vi "SPD.QE&TR Meas.vi"(5 "Progress":refnum<vi>, 6 "Temperature index":i32, 7 "Continue":refnum<vi>, 8 "Error In":errorcluster, 10 "Already done":bool, 11 "SPD.Stand Ctrl in":T1 {"spdDeviceSession"."hidSPD.Sturtup Values"."HV_bias" format="%#_6p, V"; "spdDeviceSession"."hidSPD.Sturtup Values"."TSet" format="%#_6p, DegC"; "spdDeviceSession"."hidSPD.Controller"."HV_bias" format="%#_6p, V"; "spdDeviceSession"."hidSPD.Controller"."TSet" format="%#_6p, DegC"}) -> (0 "Error Out":errorcluster, 1 "pass":bool, 2 "Report":string, 3 "SPD.Stand Ctrl out":T1 {"spdDeviceSession"."hidSPD.Sturtup Values"."HV_bias" format="%#_6p, V"; "spdDeviceSession"."hidSPD.Sturtup Values"."TSet" format="%#_6p, DegC"; "spdDeviceSession"."hidSPD.Controller"."HV_bias" format="%#_6p, V"; "spdDeviceSession"."hidSPD.Controller"."TSet" format="%#_6p, DegC"})   [LabVIEW 2018]
uses:
  typedefs/SPD.Stand Ctrl.ctl
  Instruments/SPD HID Interface/hidSPDLibForLabView/LibVIs/hidSPD Controls/hidSPD Device Session.ctl
  Instruments/SPD HID Interface/hidSPDLibForLabView/LibVIs/hidSPD Controls/hidSPD Controller.ctl
  Instruments/SPD HID Interface/hidSPDLibForLabView/LibVIs/hidSPD Controls/hidSPD SPD Type.ctl
  Instruments/KC705 DevBoard/typedefs/DevB.Session.ctl
  Instruments/KeySight 53230A/typedefs/FreqC.Session.ctl
  Instruments/KeySight 8164B/KeySight 8164B LAN InstrLib/typedefs/KeySight 8164B control.ctl
  Instruments/LeCroy SDA830/typedefs/LeCroy.Session.ctl
  typedefs/SPD.Events.ctl
  ConfigFile/SPD.Config File ctrl.ctl
  <vilib>/Utility/config.llb/Config Data RefNum.ctl
  typedefs/SPD.Meas Result.ctl
  typedefs/SPD.Queues.ctl
  typedefs/SPD.Stand state.ctl
  Instruments/KeySight 8164B/KeySight 8164B LAN InstrLib.lvlib
  <vilib>/Utility/config.llb/NI_LVConfig.lvlib
  Instruments/SPD HID Interface/hidSPDLibForLabView/hidSPDLibForLabView.lvlib
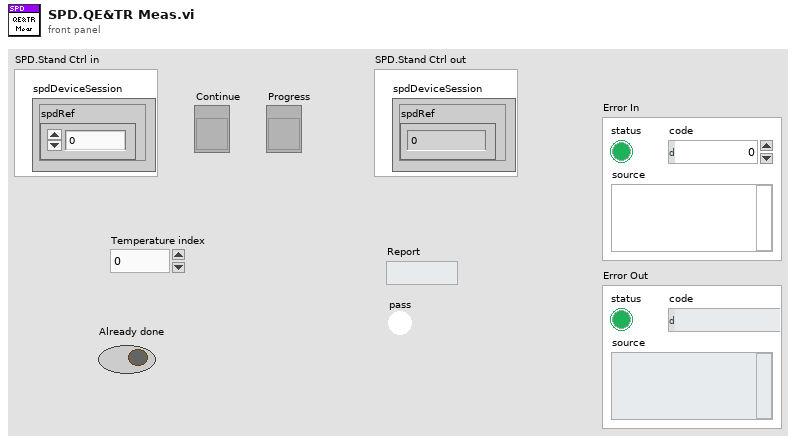
[diagram p1: front panel]
types:
  T1 = typedef "SPD.Stand Ctrl.ctl" = cluster{"spdDeviceSession":T2, "DevBSession":T5, "FreqCSession":T6, "8164BSession":T7, "LeCroySession":T8, "Events":T9, "configFile":T10, "SPD.Result":T12, "SPD.Queues":T13, "Console":refnum<vi>}
  T2 = typedef "hidSPDLibForLabView.lvlib/hidSPD Device Session.ctl" = cluster{"spdRef":u64, "connected":bool, "spdName":string, "hidSPD.Controller":T3, "hidSPD.Sturtup Values":T3, "SPD Type":T4}
  T3 = typedef "hidSPDLibForLabView.lvlib/hidSPD Controller.ctl" = cluster{"TSet":sgl, "HV_bias":sgl, "DDS_stb_code":u16}
  T4 = typedef "hidSPDLibForLabView.lvlib/hidSPD SPD Type.ctl" = enum16{"Free Run", "Gate"}
  T5 = typedef "DevB.Session.ctl" = cluster{"DevBRef":refnum<visa-resource-name>, "connected":bool}
  T6 = typedef "FreqC.Session.ctl" = cluster{"FreqCRef":refnum<visa-resource-name>, "timeout":dbl, "Gate":dbl, "connected":bool}
  T7 = typedef "KeySight 8164B LAN InstrLib.lvlib/KeySight 8164B control.ctl" = cluster{"Connection ID":refnum<k5>, "Connected":bool, "Info":string, "Slots Info":string[]}
  T8 = typedef "LeCroy.Session.ctl" = cluster{"LeCroySession":refnum<visa-resource-name>, "connected":bool}
  T9 = typedef "SPD.Events.ctl" = cluster{"DCRTest":refnum<user-event>, "Stop":refnum<user-event>}
  T10 = typedef "SPD.Config File ctrl.ctl" = cluster{"configFile ref":T11, "configFile path":path, "equipmentFile ref":T11}
  T11 = typedef "NI_LVConfig.lvlib/Config Data RefNum.ctl" = refnum<k1>
  T12 = typedef "SPD.Meas Result.ctl" = cluster{"HV_Bias":dbl[][][], "Stb_code":dbl[], "Temprature":dbl[], "Data":dbl[][][][], "DateTime":string}
  T13 = typedef "SPD.Queues.ctl" = cluster{"state queue":refnum<queue>}
  T14 = typedef "SPD.QE Test Params.ctl" = cluster{"FS":i32, "TS":i32, "Att3":dbl, "Gate":dbl, "Num Of Meas":i32, "TRStartIndex":i32, "TRRecallFile":string, "TRHistoSize":i32}
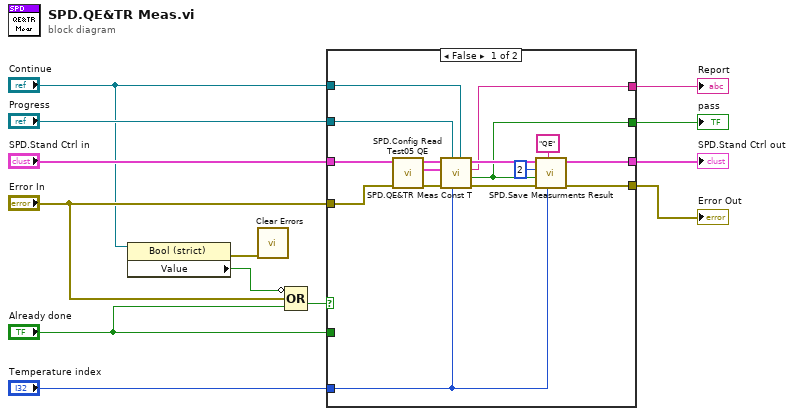
[diagram p0: block diagram]
diagram:
  n1 = property class="Bool (strict)"(reference="Continue") -> (error out=w3:errorcluster, "Value"=w2:bool)  [unwired: 1 in, 1 out]
  n2 = call <vilib>:"Clear Errors.vi"("error in (no error)"=w3) -> ()  [unwired: 5 in, 2 out]
  n3 = Compound Arithmetic op=OR(invert w2, "Error In", "Already done") -> (w6:bool)
  n4 = case shown="False" w6 {
    tunnel: [w22 w31] -> w13
    tunnel: "SPD.Stand Ctrl in" -> [w21 w32]
    tunnel: [w20 w32] -> w11
    tunnel: "Temperature index" -> [w19 _]
    tunnel: "Progress" -> [w18 _]
    tunnel: "Continue" -> [w17 _]
    tunnel: [w16 _] -> w8
    tunnel: [w14 w30] -> w7
    tunnel: "Error In" -> [w15 w31]
    tunnel: "Already done" -> [_ w30]
    frame False {
      n5 = call "SPD.Config Read Test05 QE.vi"("Error In"=w15, "SPD.Stand Ctrl in"=w21) -> ("Error Out"=w27:errorcluster, "QE Meas Params"=w26:T14, "SPD.Stand Ctrl out"=w25:T1)  [unwired: 7 in]
      n6 = call "SPD.QE&TR Meas Const T.vi"("Continue"=w17, "Temperature index"=w19, "Progress"=w18, "Error In"=w27, "QEParams"=w26, "SPD.Stand Ctrl in"=w25) -> ("Error Out"=w29:errorcluster, "pass"=w14:bool, "Report"=w16:string, "SPD.Stand Ctrl out"=w28:T1)  [unwired: 2 in]
      n7 = call "SPD.Save Measurments Result.vi"("Temperature index"=w19, "Name"="QE", "Error In"=w29, "write to file"=w14, "Param index"=2, "SPD.Stand Ctrl in"=w28) -> ("Error Out"=w22:errorcluster, "SPD.Stand Ctrl out"=w20:T1)  [unwired: 4 in]
    }
    frame True {
    }
  }
  "Error Out" <- w13
  "SPD.Stand Ctrl out" <- w11
  "Report" <- w8
  "pass" <- w7
